vi "Remove Comments Lines.vi"(8 "error in (no error)":errorcluster, 9 "Cfg Token(^#)":string="^#", 11 "CfgTable in":string[][](array[string])) -> (0 "error out":errorcluster, 3 "CfgTable out":string[][](array[string]))   [LabVIEW 2017, in "ClusterCfgTable.lvlib"]
uses:
  ClusterCfgTable.lvlib
  <userlib>/_OpenG.lib/string/string.llb/Trim Whitespace (String)__ogtk.vi
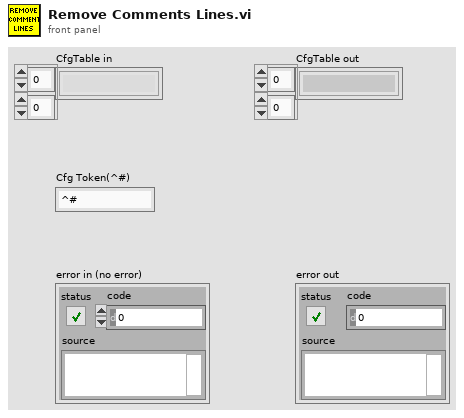
[diagram p1: front panel]
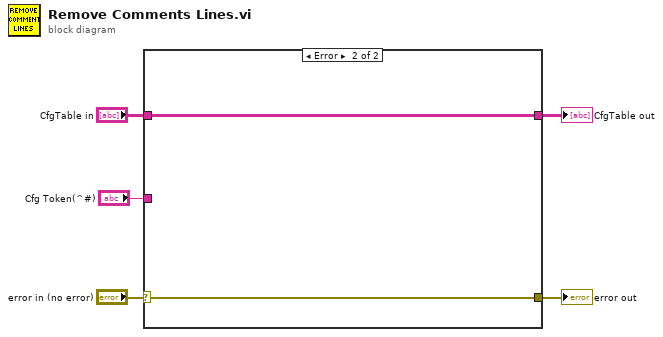
[diagram p0: block diagram]
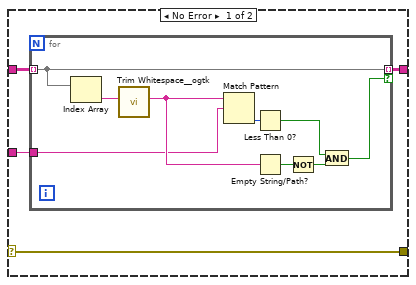
[diagram p2: hidden frame]
diagram:
  n1 = case shown="Error" "error in (no error)" {
    selector: "error in (no error)" -> [w6 w20]
    tunnel: [w9 w19] -> w5
    tunnel: "CfgTable in" -> [w8 w19]
    tunnel: "Cfg Token(^#)" -> [w7 _]
    tunnel: [w6 w20] -> w2
    frame No Error {
      n2 = for {
        tunnel: w8 -> [w18] mode=indexing
        tunnel: [w18] -> w9 mode=indexing if=w11
        tunnel: w7 -> [w10]
        n3 = Index Array(array=w18) -> (element=w17:string)  [unwired: 1 in]
        n4 = call-poly <userlib>:"Trim Whitespace__ogtk.vi"("String in"=w17) -> ("String out"=w13:string)  [unwired: 6 in]
        n5 = Match Pattern(string=w13, regular expression=w10) -> (offset past match=w16:i32)  [unwired: 1 in, 3 out]
        n6 = Less Than 0?(x=w16) -> (x < 0?=w15:bool)
        n7 = Empty String/Path?(string/path=w13) -> (empty?=w14:bool)
        n8 = Not(x=w14) -> (.not. x?=w12:bool)
        n9 = And(x=w15, y=w12) -> (x .and. y?=w11:bool)
      }
    }
    frame Error {
    }
  }
  "error out" <- w2
  "CfgTable out" <- w5
